vi "Inter_device_ops.vi"(8 "error in (no error)":errorcluster, 9 "UUT Index":i32, 10 "Comm master cluster in":T1={"Main event var"=refnum, "VIRef"=refnum, "Data path"=path "", "Reads"=0, "total number of UUT"=0, "FF refnum"={"Handle1"=0, "Handle2"=0}, "FF device id list"=[], "MODBUS resource name"="", "MODBUS Serial Parameters"={"Mode"=enum."RTU", "Default Slave Address"=0, "MODBUS timeout"=0, "Baud Rate"=0, "Parity"=0, "Flow Control"=0}, "Profibus resource name"="", "Profibus Communication ref.:"=0, "HART resource name"="", "HART long addresses (array)"=[], "Comm relay session"="", "Comm UI event"=refnum, "Write Interval (s)"=5.0, "DMM_QUEUE"=refnum, "POWER_QUEUE"=refnum, "\nTHERM_QUEUE"=refnum, "\nCOMM_QUEUE"=refnum, "TIMING_QUEUE"=refnum, "MAIN_QUEUE"=refnum, "Log path"=path ""} {"Write Interval (s)" min=0.1 max=1000.0 step=0.1}, 11 "Profibus in":refnum<class "Profibus.lvclass">) -> (0 "error out":errorcluster, 3 "Profibus out":refnum<class "Profibus.lvclass">)   [LabVIEW 2016, in "Profibus.lvclass"]
doc: "This is a vi that will do anything required when switching between devices within a cycle. For instance, Profibus requires that a new connection be made to devices with different addresses before a register is interrogated. Etc.."
uses:
  Profibus.lvclass
  MASTER_OPC.ctl
  Typedef/event var.ctl
  Typedef/Comm ui action type.ctl
  Typedef/Comm_State_enum.ctl
  Typedef/state var.ctl
  Profibus.lvclass/Profibus.ctl
  Protocol Class/Protocol.lvclass
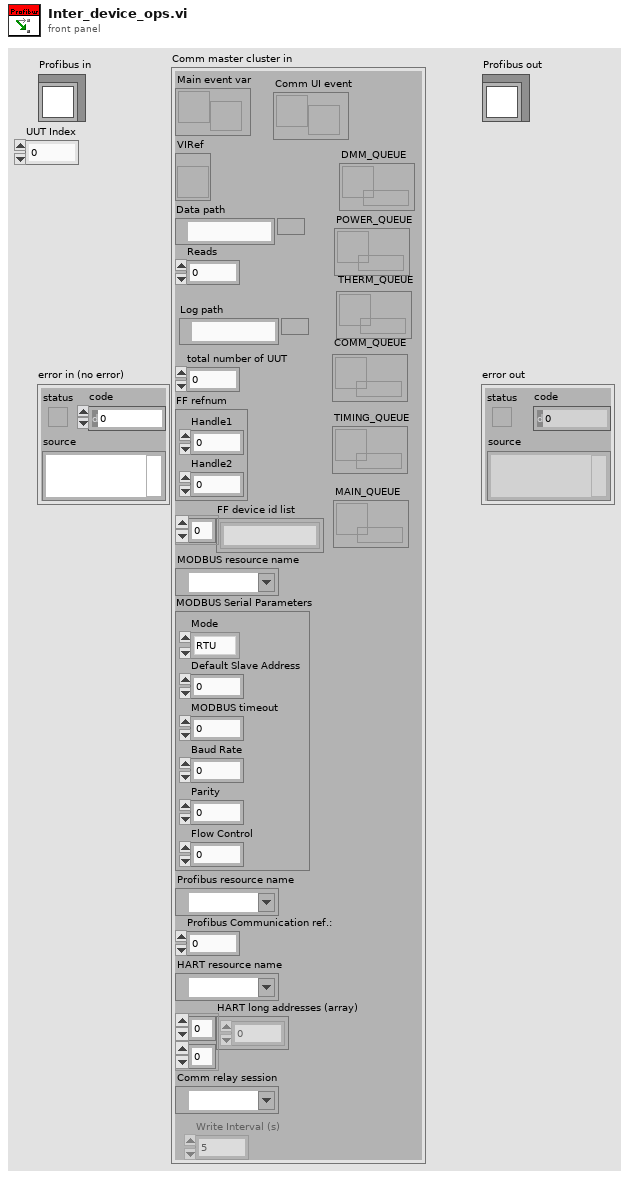
[diagram p1: front panel]
types:
  T1 = typedef "MASTER_OPC.ctl" = cluster{"Main event var":refnum<user-event>, "VIRef":refnum<vi>, "Data path":path, "Reads":i32, "total number of UUT":i32, "FF refnum":cluster{"Handle1":u32, "Handle2":u32}, "FF device id list":string[], "MODBUS resource name":refnum<visa-resource-name>, "MODBUS Serial Parameters":cluster{"Mode":enum16{"RTU", "ASCII"}, "Default Slave Address":u8, "MODBUS timeout":u32, "Baud Rate":u32, "Parity":u16, "Flow Control":u16}, "Profibus resource name":refnum<visa-resource-name>, "Profibus Communication ref.:":u8, "HART resource name":refnum<visa-resource-name>, "HART long addresses (array)":u8[][], "Comm relay session":refnum<k15>, "Comm UI event":refnum<user-event>, "Write Interval (s)":dbl, "DMM_QUEUE":refnum<queue>, "POWER_QUEUE":refnum<queue>, "\nTHERM_QUEUE":refnum<queue>, "\nCOMM_QUEUE":refnum<queue>, "TIMING_QUEUE":refnum<queue>, "MAIN_QUEUE":refnum<queue>, "Log path":path}
  T2 = typedef "CS_PB_DPV1_MSAC2_InitiateReqData.ctl" = cluster{"Communication ref.:":u8, "Send timeout:":u16, "Feat. supp. 1:":u8, "Feat. supp. 2:":u8, "Profile feat. supp. 1:":u8, "Profile feat. supp. 2:":u8, "Profile ID number:":u16, "Addional address parameter":cluster{"S-Type":bool, "S-Length:":u8, "D-Type":bool, "D-Length:":u8, "Data:":u8[]}}
  T3 = cluster{"Device address":i32, "Switch index":i32, "Communication ref.:":u8}[]
  T4 = cluster{"Device address":i32, "Switch index":i32, "Communication ref.:":u8}
  T5 = typedef "CS_PB_DPV1_MSAC2_InitiateConData.ctl" = cluster{"Communication ref.:":u8, "Remote add.:":u8, "Feat. supp. 1:":u8, "Feat. supp. 2:":u8, "Profile feat. supp. 1:":u8, "Profile feat. supp. 2:":u8, "Profile ID number:":u16, "Addional address parameter":cluster{"S-Type":bool, "S-Length:":u8, "D-Type":bool, "D-Length:":u8, "Data:":u8[]}, "Max length data unit:":u8}
  T6 = typedef "CS_PB_DPV1_MSAC2_ErrorData.ctl" = cluster{"Communication ref.:":u8, "Remote address:":u8, "Error decode:":u8, "Error code 1:":u8, "Error code 2:":u8}
  T7 = typedef "CS_PB_DPV1_MSAC2_AbortIndData.ctl" = cluster{"Remote address:":u8, "Response SAP:":u8, "Locally generated":bool, "Subnet:":u8, "Instance:":u8, "Reasoncode:":u8, "Additional detail:":u16}
  T8 = cluster{"Initiate data":T5, "Error data":T6, "Abort data":T7}
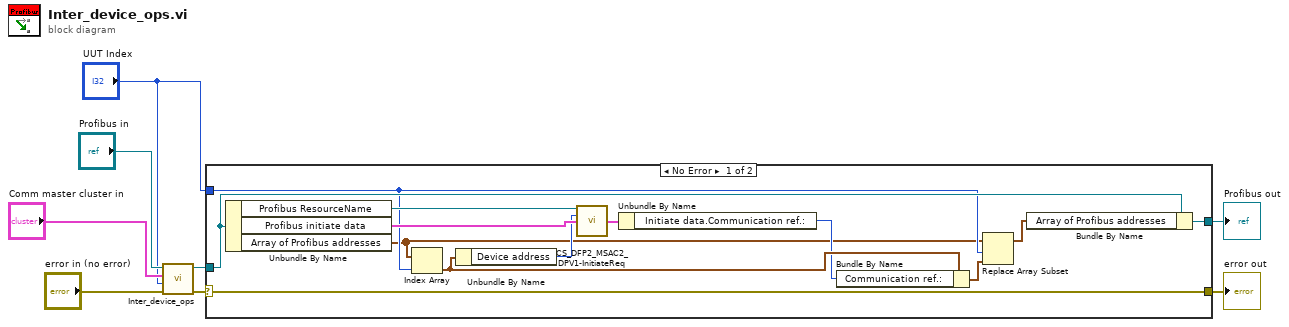
[diagram p0: block diagram]
diagram:
  n1 = call-parent "Inter_device_ops.vi"("error in (no error)"="error in (no error)", "UUT Index"="UUT Index", "Comm master cluster in"="Comm master cluster in", "Protocol in"="Profibus in") -> ("error out"=w5:errorcluster, "Protocol out"=w3:refnum<class "Profibus.lvclass">)  [unwired: 6 in]
  n2 = case shown="No Error" w5 {
    selector: w5 -> [w21 w23]
    tunnel: [w21 w23] -> w4
    tunnel: w3 -> [w16 w22]
    tunnel: [w13 w22] -> w2
    tunnel: "UUT Index" -> [w11 _]
    frame No Error {
      n3 = Unbundle By Name(w16) -> ("Profibus ResourceName"=w20:refnum<visa-resource-name>, "Profibus initiate data"=w19:T2, "Array of Profibus addresses"=w9:T3)
      n4 = Index Array(array=w9, index=w11) -> (element=w15:T4)
      n5 = Unbundle By Name(w15) -> ("Device address"=w18:i32)
      n6 = call "CS_DFP2_MSAC2_DPV1-InitiateReq.vi"("DFP2 resource name"=w20, "Profibus-Addr."=w18, "Initiate data"=w19) -> ("DPV1-Initiate"=w17:T8)  [unwired: 9 in, 3 out]
      n7 = Unbundle By Name(w17) -> ("Initiate data.Communication ref.:"=w14:u8)
      n8 = Bundle By Name(cluster=w15, "Communication ref.:"=w14) -> (w10:T4)
      n9 = Replace Array Subset(array=w9, new element=w10, index=w11) -> (w12:T3)
      n10 = Bundle By Name(cluster=w16, "Array of Profibus addresses"=w12) -> (w13:refnum<class "Profibus.lvclass">)
    }
    frame Error {
    }
  }
  "error out" <- w4
  "Profibus out" <- w2
